vi "Sequencer Main - Copy.vi"() -> ()   [LabVIEW 2018]
uses:
  EDIT Sequencer V1/Ctl/MultiColumn Sequencer Table.ctl
  Examples - 32bit/SEQUENCER/SEQUENSER v10/Sequencer v10/Ctl/Devices INI Status.ctl
  PROJEKT/NIKO/Labview/Niko V4/FTDI SPI/Ctl/Sub Addr.ctl
  <vilib>/Utility/miscctls.llb/LVRowAndColumnUnsignedTypeDef.ctl
  <vilib>/Utility/miscctls.llb/LVRowAndColumnTypeDef.ctl
  EDIT Sequencer V1/Ctl/Test Step.ctl
  EDIT Sequencer V1/Ctl/Test Result.ctl
  Ctl Main/Global Variable.vi
  EDIT Sequencer V1/Ctl/Sequencer Array.vi
  <userlib>/_OpenG.lib/file/file.llb/File Exists - Scalar__ogtk.vi
  <vilib>/Utility/config.llb/Read Key (String).vi
  <vilib>/Utility/config.llb/Read Key (U32).vi
  <vilib>/Utility/config.llb/Read Key (Double).vi
  <vilib>/Utility/config.llb/Read Key (Boolean).vi
  <vilib>/measure/madcrms.llb/Basic Averaged DC-RMS for 1 Chan.vi
  <vilib>/printing/OpenHTMLReport.llb/Open HTML Report in Browser (Refnum).vi
  <vilib>/Utility/config.llb/Write Key (I32).vi
  <vilib>/regexp/Match Regular Expression.xnode
  <vilib>/Utility/NIReport.llb/NI_report.lvclass
  <vilib>/Utility/config.llb/NI_LVConfig.lvlib
  <vilib>/Utility/NIReport.llb/NI_ReportGenerationCore.lvlib
  <vilib>/measure/NI_MAPro.lvlib
panel:
  out "Pico Scope Correction":i32
  out "Handler":u32
  out "LogMsg":string
  in  "Sequenser":u16(ring) caption="SEQUENCER" items=["", "ADB-LMS (Dowble)", "ADB-LMS (Single)", "", "", ""]
  out "System Status":T1(ring)
  in  "Operator":u16(ring) caption="OPERATOR" items=["---", "Luc Switten", "Marius Dwornic", "Ion Popesku", "Serghei Nauc", "Test SNA"]
  out "Config":string
  out "Customer":string
  out "Under Test BOARD":string caption="Test BOARD"
  out "Nom New":dbl
  out "Max New":dbl
  out "Min New":dbl
  out "Nom Old":dbl
  out "Max Old":dbl
  out "Min Old":dbl
  in  "Application Quit":bool
  in  "Tab Control Main":T2(tab)
  in  "Debug":bool
  out "File Exist?":bool
  out "Device INI Config File Path":path
  out "Dev INI OK?":bool
  in  "Dev INI":bool
  out "Box Devices":T3
  out "System INI Config File":path
  in  "Enter STEP":u32 max=1000 step=1
  in  "Barcode\nDefault":bool
  out "Cnt False All":i32
  out "Cnt Pass All":i32
  out "Cnt Total All":i32
  in  "Reset cnt":bool
  in  "Auto\nSTART":bool
  out "RETEST":bool
  out "Test Time":string
  in  "Delay 1S":bool
  in  "Tab Control Msg":T4(tab)=enum."Scope"
  in  "Msg Str":string
  out "Switch Relay Modules":T5
  out "PowSupply - GET":T6 caption="GET" {"LowerLimit" format="%#.3g"; "Upper Limit" format="%#.3g"; "Power (W)" format="%#.3g"; "Current (mA)" format="%#.3g"; "Volt (V)" format="%#.3g"}
  out "PowSupply - SET":T7 caption="SET" {"Current Limit (A)" format="%#.3g"; "Volt (V)" format="%#.3g"}
  out "Max":dbl format="%#.3g"
  out "Nominal":dbl format="%#.3g"
  out "Min":dbl format="%#.3g"
  in  "DMM Measure Monitor":T8={"Mode"=enum."*****", "Measure"="23,45V"}
  out "Limits":cluster{dbl, dbl, dbl}(slide)={1.0972762645914398, 1.2996108949416343, 0.0} caption="Limits ***" scale=0.0..200.0 scale format="%^#_4g"
  in  "Serial CMD Mon":string
  in  "Correction":i32=-8 min=-200 max=200 step=1
  in  "F-Value":dbl=0.6499999999999999 min=-1.0 max=1.0 step=0.05
  out "Measure Ch-B":T9 {"MIN Vpp" format="%#.2f"; "MAX Vpp" format="%#_2f"; "PickToPick / 2" format="%#.2f"}
  out "Measure Ch-A":T10 {"MIN Vpp" format="%#.2f"; "MAX Vpp" format="%#.2f"; "PickToPoick / 2" format="%#.2f"}
  out "Channel A":cluster{i32, dbl, dbl[]}(graph)={0, 1.9999999949504854e-06, [0.0, 0.0, 0.0, 0.0, 0.0, 0.0, 0.0, 0.0, 0.0, 0.0, 0.0, 0.0, 0.0, 0.0, 0.0, 0.0, 0.0, 0.0, 0.0, 0.0, 0.0, 0.0, 0.0, 0.0, 0.0, 0.0, 0.0, 0.0, 0.0, 0.0, 0.0, 0.0, 0.0, 0.0, 0.0, 0.0, 0.0, 0.0, 0.0, 0.0, 0.0, 0.0, 0.0, 0.0, 0.0, 0.0, 0.0, 0.0, 0.0, 0.0, 0.0, 0.0, 0.0, 0.0, 0.0, 0.0, 0.0, 0.0, 0.0, 0.0, 0.0, 0.0, 0.0, 0.0, 0.0, 0.0, 0.0, 0.0, 0.0, 0.0, 0.0, 0.0, 0.0, 0.0, 0.0, 0.0, 0.0, 0.0, 0.0, 0.0, 0.0, 0.0, 0.0, 0.0, 0.0, 0.0, 0.0, 0.0, 0.0, 0.0, 0.0, 0.0, 0.0, 0.0, 0.0, 0.0, 0.0, 0.0, 0.0, 0.0, 0.0, 0.0, 0.0, 0.0, 0.0, 0.0, 0.0, 0.0, 0.0, 0.0, 0.0, 0.0, 0.0, 0.0, 0.0, 0.0, 0.0, 0.0, 0.0, 0.0, 0.0, 0.0, 0.0, 0.0, 0.0, 0.0, 0.0, 0.0, 0.0, 0.0, 0.0, 0.0, 0.0, 0.0, 0.0, 0.0, 0.0, 0.0, 0.0, 0.0, 0.0, 0.0, 0.0, 0.0, 0.0, 0.0, 0.0, 0.0, 0.0, 0.0, 0.0, 0.0, 0.0, 0.0, 0.0, 0.0, 0.0, 0.0, 0.0, 0.0, 0.0, 0.0, 0.0, 0.0, 0.0, 0.0, 0.0, 0.0, 0.0, 0.0, 0.0, 0.0, 0.0, 0.0, 0.0, 0.0, 0.0, 0.0, 0.0, 0.0, 0.0, 0.0, 0.0, 0.0, 0.0, 0.0, 0.0, 0.0, 0.0, 0.0, 0.0, 0.0, 0.0, 0.0, 0.0, 0.0, 0.0, 0.0, 0.0, 0.0, 0.0, 0.0, 0.0, 0.0, 0.0, 0.0, 0.0, 0.0, 0.0, 0.0, 0.0, 0.0, 0.0, 0.0, 0.0, 0.0, 0.0, 0.0, 0.0, 0.0, 0.0, 0.0, 0.0, 0.0, 0.0, 0.0, 0.0, 0.0, 0.0, 0.0, 0.0, 0.0, 0.0, 0.0, 0.0, 0.0, 0.0, 0.0, 0.0, 0.0, 0.0, 0.0, 0.0, 0.0, 0.0, 0.0, 0.0, 0.0, 0.0, 0.0, 0.0, 0.0, 0.0, 0.0, 0.0, 0.0, 0.0, 0.0, 0.0, 0.0, 0.0, 0.0, 0.0, 0.0, 0.0, 0.0, 0.0, 0.0, 0.0, 0.0, 0.0, 0.0, 0.0, 0.0, 0.0, 0.0, 0.0, 0.0, 0.0, 0.0, 0.0, 0.0, 0.0, 0.0, 0.0, 0.0, 0.0, 0.0, 0.0, 0.0, 0.0, 0.0, 0.0, 0.0, 0.0, 0.0, 0.0, 0.0, 0.0, 0.0, 0.0, 0.0, 0.0, 0.0, 0.0, 0.0, 0.0, 0.0, 0.0, 0.0, 0.0, 0.0, 0.0, 0.0, 0.0, 0.0, 0.0, 0.0, 0.0, 0.0, 0.0, 0.0, 0.0, 0.0, 0.0, 0.0, 0.0, 0.0, 0.0, 0.0, 0.0, 0.0, 0.0, 0.0, 0.0, 0.0, 0.0, 0.0, 0.0, 0.0, 0.0, 0.0, 0.0, 0.0, 0.0, 0.0, 0.0, 0.0, 0.0, 0.0, 0.0, 0.0, 0.0, 0.0, 0.0, 0.0, 0.0, 0.0, 0.0, 0.0, 0.0, 0.0, 0.0, 0.0, 0.0, 0.0, 0.0, 0.0, 0.0, 0.0, 0.0, 0.0, 0.0, 0.0, 0.0, 0.0, 0.0, 0.0, 0.0, 0.0, 0.0, 0.0, 0.0, 0.0, 0.0, 0.0, 0.0, 0.0, 0.0, 0.0, 0.0, 0.0, 0.0, 0.0, 0.0, 0.0, 0.0, 0.0, 0.0, 0.0, 0.0, 0.0, 0.0, 0.0, 0.0, 0.0, 0.0, 0.0, 0.0, 0.0, 0.0, 0.0, 0.0, 0.0, 0.0, 0.0, 0.0, 0.0, 0.0, 0.0, 0.0, 0.0, 0.0, 0.0, 0.0, 0.0, 0.0, 0.0, 0.0, 0.0, 0.0, 0.0, 0.0, 0.0, 0.0, 0.0, 0.0, 0.0, 0.0, 0.0, 0.0, 0.0, 0.0, 0.0, 0.0, 0.0, 0.0, 0.0, 0.0, 0.0, 0.0, 0.0, 0.0, 0.0, 0.0, 0.0, 0.0, 0.0, 0.0, 0.0, 0.0, 0.0, 0.0, 0.0, 0.0, 0.0, 0.0, 0.0, 0.0, 0.0, 0.0, 0.0, 0.0, 0.0, 0.0, 0.0, 0.0, 0.0, 0.0, 0.0, 0.0, 0.0, 0.0, 0.0, 0.0, 0.0, 0.0, 0.0, 0.0, 0.0, 0.0, 0.0, 0.0, 0.0, 0.0, 0.0, 0.0, 0.0, 0.0, 0.0, 0.0, 0.0, 0.0, 0.0, 0.0, 0.0, 0.0, 0.0, 0.0, 0.0, 0.0, 0.0, 0.0, 0.0, 0.0, 0.0, 0.0, 0.0, 0.0, 0.0, 0.0, 0.0, 0.0, 0.0, 0.0, 0.0, 0.0, 0.0, 0.0, 0.0, 0.0, 0.0, 0.0, 0.0, 0.0, 0.0, 0.0, 0.0, 0.0, 0.0, 0.0, 0.0, 0.0, 0.0, 0.0, 0.0, 0.0, 0.0, 0.0, 0.0, 0.0, 0.0, 0.0, 0.0, 0.0, 0.0, 0.0, 0.0, 0.0, 0.0, 0.0, 0.0, 0.0, 0.0, 0.0, 0.0, 0.0, 0.0, 0.0, 0.0, 0.0, 0.0, 0.0, 0.0, 0.0, 0.0, 0.0, 0.0, 0.0, 0.0, 0.0, 0.0, 0.0, 0.0, 0.0, 0.0, 0.0, 0.0, 0.0, 0.0, 0.0, 0.0, 0.0, 0.0, 0.0, 0.0, 0.0, 0.0, 0.0, 0.0, 0.0, 0.0, 0.0, 0.0, 0.0, 0.0, 0.0, 0.0, 0.0, 0.0, 0.0, 0.0, 0.0, 0.0, 0.0, 0.0, 0.0, 0.0, 0.0, 0.0, 0.0, 0.0, 0.0, 0.0, 0.0, 0.0, 0.0, 0.0, 0.0, 0.0, 0.0, 0.0, 0.0, 0.0, 0.0, 0.0, 0.0, 0.0, 0.0, 0.0, 0.0, 0.0, 0.0, 0.0, 0.0, 0.0, 0.0, 0.0, 0.0, 0.0, 0.0, 0.0, 0.0, 0.0, 0.0, 0.0, 0.0, 0.0, 0.0, 0.0, 0.0, 0.0, 0.0, 0.0, 0.0, 0.0, 0.0, 0.0, 0.0, 0.0, 0.0, 0.0, 0.0, 0.0, 0.0, 0.0, 0.0, 0.0, 0.0, 0.0, 0.0, 0.0, 0.0, 0.0, 0.0, 0.0, 0.0, 0.0, 0.0, 0.0, 0.0, 0.0, 0.0, 0.0, 0.0, 0.0, 0.0, 0.0, 0.0, 0.0, 0.0, 0.0, 0.0, 0.0, 0.0, 0.0, 0.0, 0.0, 0.0, 0.0, 0.0, 0.0, 0.0, 0.0, 0.0, 0.0, 0.0, 0.0, 0.0, 0.0, 0.0, 0.0, 0.0, 0.0, 0.0, 0.0, 0.0, 0.0, 0.0, 0.0, 0.0, 0.0, 0.0, 0.0, 0.0, 0.0, 0.0, 0.0, 0.0, 0.0, 0.0, 0.0, 0.0, 0.0, 0.0, 0.0, 0.0, 0.0, 0.0, 0.0, 0.0, 0.0, 0.0, 0.0, 0.0, 0.0, 0.0, 0.0, 0.0, 0.0, 0.0, 0.0, 0.0, 0.0, 0.0, 0.0, 0.0, 0.0, 0.0, 0.0, 0.0, 0.0, 0.0, 0.0, 0.0, 0.0, 0.0, 0.0, 0.0, 0.0, 0.0, 0.0, 0.0, 0.0, 0.0, 0.0, 0.0, 0.0, 0.0, 0.0, 0.0, 0.0, 0.0, 0.0, 0.0, 0.0, 0.0, 0.0, 0.0, 0.0, 0.0, 0.0, 0.0, 0.0, 0.0, 0.0, 0.0, 0.0, 0.0, 0.0, 0.0, 0.0, 0.0, 0.0, 0.0, 0.0, 0.0, 0.0, 0.0, 0.0, 0.0, 0.0, 0.0, 0.0, 0.0, 0.0, 0.0, 0.0, 0.0, 0.0, 0.0, 0.0, 0.0, 0.0, 0.0, 0.0, 0.0, 0.0, 0.0, 0.0, 0.0, 0.0, 0.0, 0.0, 0.0, 0.0, 0.0, 0.0, 0.0, 0.0, 0.0, 0.0, 0.0, 0.0, 0.0, 0.0, 0.0, 0.0, 0.0, 0.0, 0.0, 0.0, 0.0, 0.0, 0.0, 0.0, 0.0, 0.0, 0.0, 0.0, 0.0, 0.0, 0.0, 0.0, 0.0, 0.0, 0.0, 0.0, 0.0, 0.0, 0.0, 0.0, 0.0, 0.0, 0.0, 0.0, 0.0, 0.0, 0.0, 0.0, 0.0, 0.0, 0.0, 0.0, 0.0, 0.0, 0.0, 0.0, 0.0, 0.0, 0.0, 0.0, 0.0, 0.0, 0.0, 0.0, 0.0, 0.0, 0.0, 0.0, 0.0, 0.0, 0.0, 0.0, 0.0, 0.0, 0.0, 0.0, 0.0, 0.0, 0.0, 0.0, 0.0, 0.0, 0.0, 0.0, 0.0, 0.0, 0.0, 0.0, 0.0, 0.0, 0.0, 0.0, 0.0, 0.0, 0.0, 0.0, 0.0, 0.0, 0.0, 0.0, 0.0, 0.0, 0.0, 0.0, 0.0, 0.0, 0.0, 0.0, 0.0, 0.0, 0.0, 0.0, 0.0, 0.0, 0.0, 0.0, 0.0, 0.0, 0.0, 0.0, 0.0, 0.0, 0.0, 0.0, 0.0, 0.0, 0.0, 0.0, 0.0, 0.0, 0.0, 0.0, 0.0, 0.0, 0.0, 0.0, 0.0, 0.0, 0.0, 0.0, 0.0, 0.0, 0.0, 0.0, 0.0, 0.0, 0.0, 0.0, 0.0, 0.0, 0.0, 0.0, 0.0, 0.0, 0.0, 0.0, 0.0, 0.0]}
  out "Channel B":cluster{i32, dbl, dbl[]}(graph)={0, 1.9999999949504854e-06, [0.0, 0.03891109958189642, 0.03891109958189642, 0.0, 0.03891109958189642, 0.03891109958189642, 0.03891109958189642, 0.0, 0.0, 0.03891109958189642, 0.03891109958189642, 0.03891109958189642, 0.03891109958189642, -0.03891109958189642, 0.0, 0.0, 0.0, 0.03891109958189642, 0.0, 0.0, 0.03891109958189642, 0.0, 0.03891109958189642, 0.0, 0.0, 0.0, 0.0, 0.03891109958189642, 0.03891109958189642, 0.0, -0.03891109958189642, 0.03891109958189642, 0.0, 0.03891109958189642, 0.03891109958189642, 0.03891109958189642, 0.0, 0.0, 0.03891109958189642, 0.0, 0.0, 0.03891109958189642, 0.03891109958189642, 0.0, 0.0, 0.03891109958189642, 0.0, 0.03891109958189642, 0.0, 0.0, 0.0, 0.03891109958189642, 0.03891109958189642, 0.0, 0.0, 0.0, 0.03891109958189642, 0.03891109958189642, 0.0, 0.0, 0.03891109958189642, 0.0, 0.0, -0.03891109958189642, 0.03891109958189642, 0.0, 0.0, 0.0, 0.0, 0.03891109958189642, 0.0, 0.0, 0.03891109958189642, 0.0, 0.03891109958189642, -0.03891109958189642, 0.0, 0.0, 0.03891109958189642, 0.0, 0.03891109958189642, 0.03891109958189642, 0.0, 0.0, 0.03891109958189642, 0.0, 0.03891109958189642, 0.0, 0.0, 0.0, 0.0, 0.03891109958189642, 0.0, 0.0, 0.03891109958189642, 0.03891109958189642, 0.0, 0.0, 0.0, 0.03891109958189642, 0.0, 0.0, 0.0, 0.0, 0.0, 0.0, 0.0, 0.0, 0.0, 0.0, 0.0, 0.03891109958189642, 0.0, 0.03891109958189642, 0.03891109958189642, 0.0, 0.03891109958189642, 0.03891109958189642, 0.0, 0.03891109958189642, 0.0, 0.0, 0.0, 0.03891109958189642, 0.03891109958189642, 0.0, 0.0, 0.0, 0.0, 0.0, 0.03891109958189642, 0.0, 0.03891109958189642, 0.0, 0.0, 0.03891109958189642, 0.03891109958189642, 0.0, 0.0, 0.0, 0.03891109958189642, 0.03891109958189642, 0.0, 0.0, 0.03891109958189642, 0.0, 0.0, 0.03891109958189642, 0.0, 0.0, 0.0, 0.03891109958189642, 0.0, 0.03891109958189642, 0.03891109958189642, 0.03891109958189642, 0.03891109958189642, 0.03891109958189642, 0.0, 0.0, 0.0, 0.03891109958189642, 0.03891109958189642, 0.03891109958189642, 0.03891109958189642, 0.03891109958189642, 0.0, 0.03891109958189642, 0.0, 0.0, 0.0, 0.03891109958189642, 0.0, 0.03891109958189642, 0.0, 0.0, 0.0, 0.0, 0.03891109958189642, 0.0, 0.0, 0.03891109958189642, 0.0, 0.03891109958189642, 0.03891109958189642, 0.0, 0.03891109958189642, 0.0, 0.03891109958189642, 0.03891109958189642, 0.03891109958189642, 0.03891109958189642, 0.0, 0.03891109958189642, 0.03891109958189642, 0.0, 0.0, 0.03891109958189642, 0.03891109958189642, 0.03891109958189642, 0.03891109958189642, 0.0, 0.0, 0.0, 0.0, 0.03891109958189642, 0.0, 0.03891109958189642, 0.0, 0.03891109958189642, 0.0, 0.0, 0.0, 0.03891109958189642, 0.03891109958189642, 0.0, 0.0, 0.0, 0.0, 0.03891109958189642, 0.0, 0.0, 0.0, 0.0, 0.03891109958189642, 0.03891109958189642, 0.03891109958189642, 0.0, 0.03891109958189642, 0.0, 0.0, 0.0, 0.03891109958189642, 0.03891109958189642, 0.03891109958189642, 0.03891109958189642, 0.0, 0.0, 0.0, 0.0, 0.03891109958189642, 0.03891109958189642, 0.03891109958189642, 0.03891109958189642, 0.0, 0.0, 0.0, 0.0, 0.0, 0.0, 0.03891109958189642, 0.0, 0.0, 0.0, -0.03891109958189642, 0.0, 0.0, 0.03891109958189642, 0.03891109958189642, 0.0, 0.0, 0.03891109958189642, 0.03891109958189642, 0.0, 0.0, 0.03891109958189642, -0.03891109958189642, 0.03891109958189642, 0.03891109958189642, 0.0, 0.0, 0.0, 0.0, 0.03891109958189642, 0.03891109958189642, 0.0, 0.03891109958189642, 0.0, 0.0, 0.0, 0.0, 0.0, 0.0, 0.0, 0.03891109958189642, 0.03891109958189642, 0.0, 0.03891109958189642, 0.03891109958189642, 0.0, 0.0, 0.0, 0.03891109958189642, 0.0, 0.0, 0.0, 0.0, 0.0, 0.0, 0.0, 0.0, 0.0, 0.0, 0.03891109958189642, 0.0, 0.0, 0.0, 0.0, 0.0, 0.0, 0.0, 0.03891109958189642, 0.0, 0.0, 0.0, 0.0, 0.0, 0.0, 0.0, 0.0, 0.0, 0.03891109958189642, 0.0, 0.0, 0.0, 0.03891109958189642, 0.0, 0.03891109958189642, 0.0, 0.03891109958189642, 0.03891109958189642, 0.0, 0.03891109958189642, 0.0, 0.03891109958189642, 0.0, 0.03891109958189642, 0.0, 0.03891109958189642, 0.0, -0.03891109958189642, 0.0, 0.0, 0.0, 0.0, 0.0, 0.03891109958189642, 0.0, 0.03891109958189642, 0.0, 0.03891109958189642, 0.03891109958189642, 0.0, 0.0, 0.0, 0.03891109958189642, 0.0, 0.03891109958189642, 0.03891109958189642, 0.0, 0.0, 0.0, 0.0, 0.0, 0.0, 0.03891109958189642, 0.03891109958189642, 0.0, 0.0, 0.0, 0.0, 0.0, 0.0, 0.0, -0.03891109958189642, 0.03891109958189642, 0.0, 0.03891109958189642, 0.03891109958189642, 0.0, 0.0, 0.03891109958189642, 0.0, 0.03891109958189642, 0.0, 0.0, 0.03891109958189642, 0.03891109958189642, 0.03891109958189642, 0.0, 0.0, 0.03891109958189642, 0.03891109958189642, 0.03891109958189642, 0.0, 0.0, 0.0, 0.0, 0.0, 0.0, 0.0, 0.0, 0.03891109958189642, 0.0, 0.03891109958189642, 0.0, 0.0, 0.03891109958189642, 0.03891109958189642, 0.03891109958189642, 0.0, 0.0, 0.0, 0.0, 0.03891109958189642, -0.03891109958189642, 0.03891109958189642, 0.0, 0.03891109958189642, 0.03891109958189642, 0.0, 0.0, 0.03891109958189642, 0.0, 0.0, 0.03891109958189642, 0.0, 0.0, 0.0, -0.03891109958189642, 0.03891109958189642, 0.03891109958189642, 0.03891109958189642, 0.03891109958189642, 0.03891109958189642, 0.03891109958189642, 0.03891109958189642, 0.0, 0.0, 0.0, 0.0, 0.0, 0.0, 0.0, 0.0, 0.03891109958189642, 0.03891109958189642, 0.0, 0.0, 0.0, 0.03891109958189642, 0.03891109958189642, 0.0, 0.0, 0.0, 0.03891109958189642, 0.0, 0.0, 0.0, 0.0, 0.0, 0.03891109958189642, 0.03891109958189642, 0.03891109958189642, 0.0, 0.0, 0.0, 0.03891109958189642, 0.0, 0.03891109958189642, 0.03891109958189642, 0.03891109958189642, 0.03891109958189642, 0.0, 0.03891109958189642, 0.0, 0.0, 0.0, 0.03891109958189642, 0.0, 0.0, 0.0, 0.0, 0.0, 0.03891109958189642, 0.03891109958189642, 0.03891109958189642, 0.0, 0.0, 0.03891109958189642, 0.03891109958189642, -0.03891109958189642, 0.0, 0.03891109958189642, 0.0, 0.0, 0.0, 0.03891109958189642, 0.03891109958189642, 0.0, 0.0, 0.0, 0.0, 0.0, 0.0, 0.0, 0.0, 0.03891109958189642, 0.03891109958189642, 0.03891109958189642, 0.0, 0.03891109958189642, 0.03891109958189642, 0.03891109958189642, 0.0, 0.03891109958189642, 0.0, 0.0, 0.03891109958189642, 0.0, 0.03891109958189642, 0.0, 0.0, 0.0, 0.0, 0.0, 0.0, 0.0, 0.0, 0.03891109958189642, 0.0, 0.03891109958189642, 0.03891109958189642, 0.03891109958189642, 0.03891109958189642, 0.0, 0.03891109958189642, 0.03891109958189642, 0.0, 0.0, 0.0, 0.03891109958189642, 0.0, 0.03891109958189642, 0.03891109958189642, 0.0, 0.0, 0.0, 0.0, 0.0, 0.0, 0.03891109958189642, 0.0, 0.0, 0.03891109958189642, 0.03891109958189642, 0.0, 0.0, 0.0, 0.0, 0.03891109958189642, 0.03891109958189642, 0.0, 0.0, 0.0, 0.03891109958189642, 0.0, 0.0, 0.0, 0.0, 0.03891109958189642, 0.0, 0.0, 0.0, 0.0, 0.03891109958189642, 0.03891109958189642, 0.03891109958189642, 0.0, 0.0, 0.0, 0.03891109958189642, 0.03891109958189642, 0.03891109958189642, 0.0, 0.03891109958189642, 0.0, 0.0, 0.0, 0.0, 0.03891109958189642, 0.0, 0.03891109958189642, 0.0, 0.0, 0.03891109958189642, 0.03891109958189642, 0.03891109958189642, 0.0, 0.0, 0.03891109958189642, 0.0, 0.0, 0.03891109958189642, 0.0, 0.0, 0.03891109958189642, 0.03891109958189642, 0.0, 0.03891109958189642, 0.0, 0.0, 0.0, 0.0, 0.0, 0.0, 0.0, 0.03891109958189642, 0.03891109958189642, 0.0, 0.03891109958189642, 0.0, 0.03891109958189642, 0.0, 0.0, 0.03891109958189642, 0.03891109958189642, 0.0, 0.03891109958189642, 0.03891109958189642, -0.03891109958189642, 0.03891109958189642, 0.0, 0.03891109958189642, 0.0, -0.03891109958189642, 0.0, 0.03891109958189642, 0.03891109958189642, 0.03891109958189642, 0.0, 0.0, 0.0, 0.0, 0.0, 0.03891109958189642, 0.0, 0.03891109958189642, 0.0, 0.0, 0.0, 0.0, 0.03891109958189642, 0.0, 0.03891109958189642, 0.0, 0.03891109958189642, 0.0, 0.03891109958189642, 0.0, 0.03891109958189642, 0.0, 0.03891109958189642, 0.0, 0.03891109958189642, 0.0, 0.03891109958189642, 0.0, 0.0, 0.03891109958189642, 0.0, 0.03891109958189642, 0.0, 0.0, 0.0, 0.0, 0.0, 0.0, 0.03891109958189642, 0.0, 0.0, 0.03891109958189642, 0.0, 0.03891109958189642, 0.0, 0.0, 0.0, 0.0, 0.0, 0.03891109958189642, 0.03891109958189642, 0.0, -0.03891109958189642, 0.0, 0.03891109958189642, 0.0, 0.0, 0.03891109958189642, 0.03891109958189642, 0.0, 0.03891109958189642, 0.03891109958189642, 0.03891109958189642, 0.0, 0.03891109958189642, 0.03891109958189642, 0.03891109958189642, 0.0, 0.0, 0.03891109958189642, 0.03891109958189642, 0.03891109958189642, 0.03891109958189642, 0.0, 0.03891109958189642, 0.0, 0.0, 0.0, 0.03891109958189642, 0.03891109958189642, 0.03891109958189642, 0.0, 0.0, 0.03891109958189642, 0.0, 0.0, 0.03891109958189642, 0.0, 0.03891109958189642, 0.0, 0.03891109958189642, 0.0, 0.03891109958189642, 0.0, 0.0, 0.0, 0.0, 0.0, 0.03891109958189642, 0.0, 0.0, 0.0, 0.0, 0.03891109958189642, 0.0, 0.0, 0.0, 0.0, 0.0, 0.0, 0.0, 0.0, 0.0, 0.0, 0.0, 0.0, 0.03891109958189642, -0.03891109958189642, 0.03891109958189642, 0.0, 0.07782219916379284, 0.03891109958189642, 0.0, 0.03891109958189642, 0.0, 0.03891109958189642, 0.0, 0.03891109958189642, 0.03891109958189642, 0.03891109958189642, 0.03891109958189642, 0.03891109958189642, 0.0, 0.0, 0.03891109958189642, 0.0, 0.03891109958189642, 0.0, 0.0, 0.0, 0.0, 0.0, 0.03891109958189642, 0.03891109958189642, 0.0, 0.0, 0.03891109958189642, 0.03891109958189642, 0.03891109958189642, 0.0, 0.03891109958189642, 0.0, 0.03891109958189642, 0.03891109958189642, 0.0, 0.03891109958189642, -0.03891109958189642, 0.0, 0.03891109958189642, 0.0, 0.03891109958189642, 0.03891109958189642, 0.0, 0.03891109958189642, 0.0, 0.0, 0.0, 0.0, 0.0, 0.03891109958189642, 0.0, 0.0, 0.0, 0.03891109958189642, 0.07782219916379284, 0.0, 0.03891109958189642, 0.0, 0.0, 0.03891109958189642, 0.0, 0.0, 0.03891109958189642, 0.0, 0.03891109958189642, 0.0, 0.03891109958189642, 0.0, 0.0, 0.03891109958189642, 0.0, 0.0, 0.03891109958189642, 0.0, 0.03891109958189642, 0.0, 0.0, 0.0, 0.03891109958189642, 0.03891109958189642, 0.03891109958189642, -0.03891109958189642, 0.03891109958189642, 0.03891109958189642, 0.03891109958189642, 0.03891109958189642, 0.0, 0.0, 0.0, 0.0, 0.0, 0.03891109958189642, 0.0, 0.0, 0.0, 0.0, 0.03891109958189642, 0.0, 0.0, 0.0, 0.03891109958189642, 0.03891109958189642, 0.0, 0.0, 0.03891109958189642, 0.0, 0.03891109958189642, 0.03891109958189642, 0.0, 0.0, 0.0, 0.03891109958189642, 0.03891109958189642, 0.0, 0.03891109958189642, 0.0, 0.0, 0.0, 0.03891109958189642, 0.03891109958189642, 0.0, 0.0, 0.03891109958189642, 0.03891109958189642, 0.03891109958189642, 0.03891109958189642, 0.03891109958189642, 0.03891109958189642, 0.03891109958189642, 0.03891109958189642, 0.0, 0.0, 0.03891109958189642, 0.03891109958189642, 0.0, 0.0, 0.03891109958189642, 0.03891109958189642, 0.0, 0.03891109958189642, 0.0, 0.03891109958189642, 0.03891109958189642, 0.0, 0.03891109958189642, 0.0, 0.0, 0.0, 0.0, 0.03891109958189642, 0.0, 0.0, 0.03891109958189642, 0.03891109958189642, 0.0, 0.07782219916379284, 0.0, 0.0, 0.03891109958189642, 0.0, 0.03891109958189642, 0.0, 0.03891109958189642, 0.03891109958189642, 0.0, 0.0, 0.0, 0.0, 0.0, 0.03891109958189642, 0.03891109958189642, 0.03891109958189642, 0.03891109958189642, 0.0, 0.0, 0.03891109958189642, 0.0, 0.0, 0.03891109958189642, 0.0, 0.0, 0.03891109958189642, 0.03891109958189642, 0.03891109958189642, 0.0, 0.03891109958189642, 0.0, 0.0, 0.0, 0.03891109958189642, 0.03891109958189642, 0.03891109958189642, 0.03891109958189642, 0.03891109958189642, 0.0, 0.0, 0.0, 0.0, 0.0, 0.0, 0.03891109958189642, 0.03891109958189642, 0.0, 0.03891109958189642, 0.03891109958189642, 0.0, 0.03891109958189642, -0.03891109958189642, 0.03891109958189642, 0.0, 0.03891109958189642, 0.0, -0.03891109958189642, 0.0, 0.03891109958189642, 0.0, 0.0, 0.03891109958189642, 0.03891109958189642, 0.03891109958189642, 0.03891109958189642, 0.03891109958189642, 0.07782219916379284, 0.03891109958189642, 0.0, 0.03891109958189642, 0.0, 0.03891109958189642, 0.0, 0.03891109958189642, 0.03891109958189642, 0.03891109958189642, 0.03891109958189642, 0.0, 0.0, 0.0, 0.03891109958189642, 0.0, 0.03891109958189642, 0.03891109958189642]}
  in  "Delay":u16=2 max=10 step=1
  in  "Tab Edit/Run":enum32{"Edit", "Run"}(tab)
  in  "Test Squencer Edit":T11
  in  "Test Sequencer Run":T11
  in  "Dig-IN Claster":T12
  in  "Break Point Line":u32
  out "Sys Err":bool
  in  "Report Auto":bool=TRUE
  in  "Break On First Err":bool=TRUE caption="Break On\n3x First Err"
  in  "Button Create Report":bool
  in  "Abort Test":bool
  in  "Run Test":bool
  in  "Button Retest":bool
  in  "Button Next Step":bool caption="Next Step"
  in  "Debugging":bool
  in  "Edit Sequenser":bool
  out "Cnt False":i32
  out "Cnt Pass":i32
  out "Cnt Total":i32
  out "Gen Test Status":bool
  in  "Load Sequenser":bool
  in  "Message":string="..."
  in  "Barcode":string="ADB-12345"
  out "Date Time":string
  in  "Auto\nRestart":u16=1 min=1 max=99
  out "Restart Cnt":u16
  out "Auto\nReStart":bool
  in  "WebBrowser":refnum<k7>(container)
  in  "Open in Default IE":bool
  out "Help":string="GPIO-Out Set RELAY Modules: \n(Step-Id = 10)                        std_logic_vector(9 downto 0) use (9 downto 0)\n      0>1>d:1                          --set single decimal channel ;\n      0>1>b:0000110001       -- set binary multiple channels ;\n      0>1>s:0000000011        -- Set  binary (only 1 channels) ;\n      0>1>r:0000000011        -- Reset  binary (only 1 channels) ;\n      --option 'Togle Channel' not in use\n\nGPIO-Out Set SYSTEM: \n(Step-Id = 11)                           std_logic_vector(9 downto 0) use (3 downto 0)\n      0>1>b:0000110001        -- set binary multiple channels ;\n\nRESET Modules ( (GPIO->ON) >> (GPIO->OFF) )\n(Step-Id = 12)\n    0>1>rst:0000000011>250>1000        -- reset 0>1>channel:xx>Delay(Active)>Delay(Passive)\n\nDELAY (mS)\n(Step-Id = 13)\n    750                                     --Delay (750mS)\n\nPOWER SUPPLY (BK9201) \n   1- Set (Step-Id = 15)\n        57,0>0,2>ON           --set Volt>Current>ON/OFF\n\n   2- Get (Step-Id = 16)\n       Volt?\n       Current?\n       Power?\n\nDMM bk5492C\n(Step-Id = 20)                   <measure DMM-DC Volt>\n       V-DC>0                   --Auto Range\n       V-DC>0,1                --Manual Range (0,1 1 10 100 1000)V\n       -----------------------------------------------------------------------------------------------\n                                          <measure DMM-AC Volt>\n       V-AC>0                   --Auto Range\n       V-AC>0,1                --Manual Range (0,1 1 10 100 750)V\n       -----------------------------------------------------------------------------------------------\n                                                               <measure DMM-Resistors 2x Wires>\n       R-2W>0                 --Auto Range\n           R-2W>1M              --Manual Range (10, 100, 1K, 10K, 100K, 1M, 10M, 100M)\n       ----------------------------------------------------------------------------------------------- \n                                                               <measure DMM-Resistors 4x Wires>\n       R-4W>0                 --Auto Range\n           R-4W>10K             --Manual Range (10, 100, 1K, 10K, 100K, 1M, 10M, 100M)  \n       -----------------------------------------------------------------------------------------------\n\n      >false:100:2       --in case of a FALSE, repeat test 2x times, gump to step100\n\nFLASH ADB\n(Step-Id = 70)\n       adb_flash.bat      --xxxx.bat -name of bat file, location at ..\\FLASH\n\nSERIAL CMD (RS232)\n(Step-Id = 60) \n       >>open;<firmware version>      --Open Serial COM and check firmware version\n\n      >false:100:2       --in case of a FALSE, repeat test 2x times, gump to step100\n\n\nBLUETOOTH (u-blox)\n(Step-Id = 40)                   <Connect To ADB Bloetooth Interfice>\n\nRFID (Arduino & Sparkfun uno)\n(Step-Id = 45)                   <Connect To ADB RFID Interfice>\n      >false:100:2       --in case of a FALSE, repeat test 2x times, gump to step100\n\nRFID (Arduino & Sparkfun uno)\n(Step-Id = 46)                   <Connect To ADB RFID Interfice>\n      >false:100:2       --in case of a FALSE, repeat test 2x times, gump to step100\n\nPicoScope (SET)\n(Step-Id = 51)             --Set PicoScope (Time Aut = 2000mS)\n      A>8000>1000           Channel <A, B> ; Sampels ;TimeBase\n\nPicoScope (GET)\n(Step-Id = 51)             --Read PicoScope DATA\n      A>>false:100:2            Channel <A, B> ; Sampels ;TimeBase\n                                          --if FALSE, repeat test 2x times, gump to step100\n\n(Step-Id = 52)             --Read PicoScope (Time Aut = 2000mS)\n      B>false:46:3               Channel <A, B> if FALSE, goto step <46>, retry <3> times \n\n(Step-Id = 53)                     --Read PicoScope \"Positive / Negative Measurement\" (Time Aut = 2000mS)\n      B>Positive>false:46:3               Channel <A, B> if FALSE, goto step <46>, retry <3> times \n      B>Negative\n\n\n\n\n\n\n\n   "
  # "ELETEST-Ro Test SEQUENCER"
  # "Elemaster Romania"
  # "ver 3,0"
  # "TEST Report STATUS"
  # "Dig Sys Input"
  # "Fixture Closed"
  # "Barcode"
  # "Stop"
  # "Run"
  # "TOTAL:"
  # "Sequencer / Debugging"
  # "PASS:"
  # "FALSE:"
  # "1"
  # "2"
  # "3"
  # "4"
  # "5"
  # "6"
  # "7"
  # "8"
  # "9"
  # "10"
  # "Ch-A"
  # "Ch-B"
  # "DMM Measure Mode"
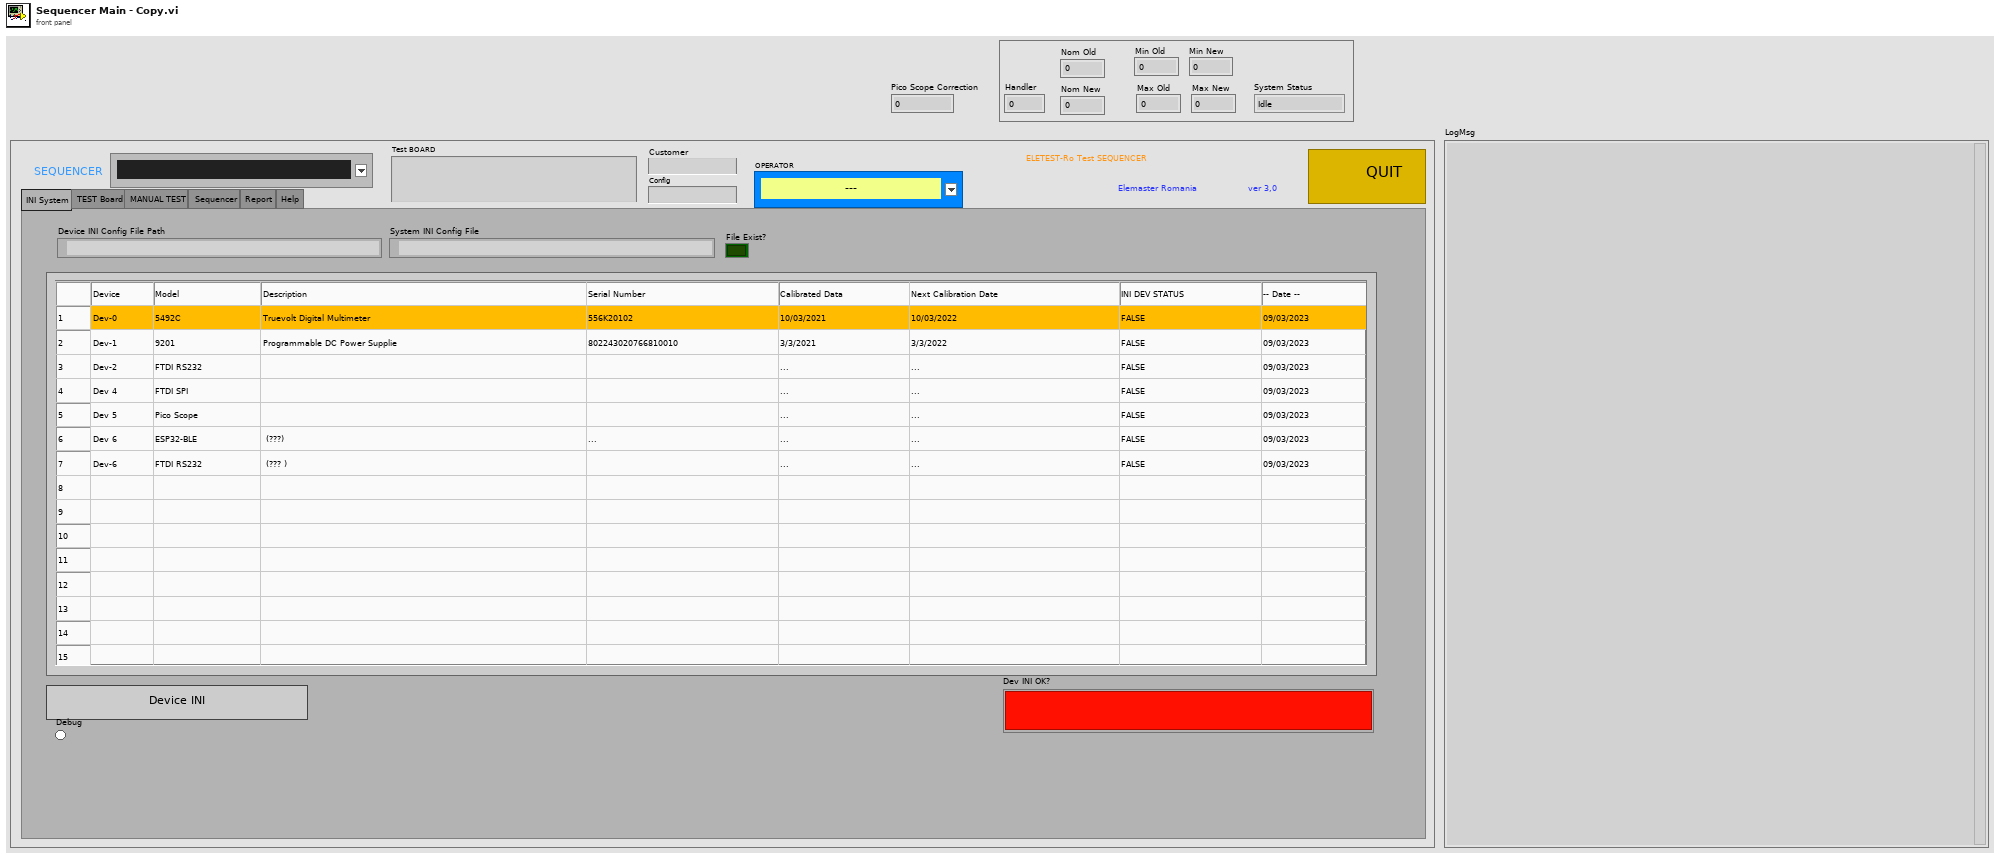
[diagram p1: front panel]
types:
  T1 = enum16{"Idle", "INI System", "INI Devices", "START Sequencer", "INI Secuencer", "Run Sequencer", "STOP Sequencer", "Report Generation", "Test Load Monitor", "QUIT"}
  T2 = enum32{"INI System", "TEST Board", "MANUAL TEST", "Sequencer ", "Report", "Help"}
  T3 = typedef "Devices INI Status.ctl" = i32
  T4 = enum32{"Msg", "Settings", "PowSupply", "DMM", "Serial", "Scope", "Bluetooth"}
  T5 = cluster{"SW 0":bool[], "SW 1":bool[], "SW 2":bool[], "SW 3":bool[], "SW 4":bool[], "SW 5":bool[], "SW 6":bool[], "SW 7":bool[], "Main Power Supplay ON/OFF":bool, "BASE":bool[][]}
  T6 = cluster{"Volt (V)":dbl, "Current (mA)":dbl, "Power (W)":dbl, "Upper Limit":dbl, "LowerLimit":dbl}
  T7 = cluster{"Volt (V)":dbl, "Current Limit (A)":dbl, "ON/OFF":bool}
  T8 = cluster{"Mode":enum16{"*****", "Voltage - DC", "Voltage - AC", "Current - DC", "Current - AC", "Diode", "Resistans 2-Wire", "Resistans 4-Wire", "Capasitor"}, "Measure":string}
  T9 = cluster{"PickToPick / 2":dbl, "MAX Vpp":dbl, "MIN Vpp":dbl}
  T10 = cluster{"PickToPoick / 2":dbl, "MAX Vpp":dbl, "MIN Vpp":dbl}
  T11 = typedef "MultiColumn Sequencer Table.ctl" = i32
  T12 = cluster{"Stop":bool, "Fixture Close":bool, "digIn 3":bool, "digIn 4":bool, "Run":bool}
  T13 = typedef "Semaphore RefNum" = refnum<k1>
  T14 = typedef "LVRowAndColumnUnsignedTypeDef.ctl" = cluster{"Row":u32, "Column":u32}
  T15 = typedef "LVRowAndColumnTypeDef.ctl" = cluster{"Row":i32, "Column":i32}
  T16 = typedef "Test Step.ctl" = cluster{"Step ID":u16, "Step Description":string, "Step Type":u16, "Test Values":cluster{"Numeric Value":dbl, "Str Value":string, "Boolean Value":bool, "Upper Limit":dbl, "Lower Limit":dbl}, "Parameters":string, "Run/Skip":bool, "Test Result":T17, "Report":bool, "Measure Units":string}
  T17 = typedef "Test Result.ctl" = enum16{"Idle", "PASS", "FALSE"}
  T18 = enum8{"Enabled", "Disabled", "Disabled and Grayed Out"}
  T19 = typedef "NI_LVConfig.lvlib/Config Data RefNum.ctl" = refnum<k1>
  T20 = typedef "Sub Addr.ctl" = u16
  T21 = enum32{"Msg", "Settings", "PowSupply", "DMM", "Serial", "Scope"}
  T22 = cluster{"ClockRate":u32, "LatencyTimer":u8, "configOptions 24-31":i8, "configOptions 16-23":i8, "configOptions 8-15":i8, "configOptions 0-7":u32, "Pin":u32, "reserved":u16}
  T23 = enum16{"Set Decimal", "Set Binary", "Set Channels", "Reset Channels"}
  T24 = enum16{"Set Decimal", "Set Binary", "Set Channels", "Reset Channels", "Togle Channel"}
  T25 = enum16{"*****", "Voltage - DC", "Voltage - AC", "Current - DC", "Current - AC", "Diode", "Resistans 2-Wire", "Resistans 4-Wire", "Capasitor"}
  T26 = cluster{"Enabled":bool, "Coupling":i16, "Range":u16, "Analogue Offset":sgl}
  T27 = cluster{"preTriggerSamples":u32, "postTriggerSamples":u32, "timebase":u32, "Down-Sample Mode":i32, "Down Sample Ratio":u32, "Oversample":i16}
  T28 = cluster{"Trigger Enabled":bool, "Trigger Source":enum16{"Channel A", "Channel B", "Channel C", "Channel D", "Ext."}, "Trigger Threshold (Volts)":dbl, "Trigger Direction":u16, "Trigger Delay (samples)":u32, "Auto Trigger Time (ms)":i16}
  T29 = cluster{"Peak-to-Peak Voltage (microvolts)":u32, "Offset Voltage (microvolts)":i32, "Wave Type":i16, "Sweep Type":i32, "Shots":u32, "Sweeps":u32, "Trigger Type":i32, "Trigger Source":i32, "Ext. Threshold (ADC count)":i16, "White Noise":bool}
  T30 = cluster{"Start Frequency":dbl, "Stop Frequency":dbl, "Increment":dbl, "Dwell Time (seconds)":dbl}
  T31 = enum16{"Standard Report", "HTML", "Word", "Excel"}
  T32 = cluster{"top":dbl, "left":dbl, "right":dbl, "bottom":dbl}
  T33 = typedef "LVStringsAndValuesArrayTypeDef_U16.ctl" = cluster{"String":string, "Value":u16}[]
  T34 = typedef "Serial_VISA.ctl" = cluster{"VISA resource name":string, "Vendor":string, "SerialNumber":string, "CalibrationTime":string, "Dev Ok":bool, "Model":string, "Next CalibrationTime":string}
  T35 = cluster{"Driver Version":string, "USB Version":string, "Hardware":string, "Variant":string, "Batch and Serial":string, "Cal Date":string, "Kernel Version":string, "Digital HW Version":string, "Analogue HW Version":string, "Firmware 1":string, "Firmware 2":string, "MSO":bool, "Number of Channels":i16}
  T36 = cluster{"Lower Limit":dbl, "Upper Limit":dbl, "Numeric Value":dbl}
  T37 = cluster{"Lower Limit":dbl, "Upper Limit":dbl, "Result Value":dbl}
diagram:
  n1 = in-place {
    in-place-border: [w7] -> w1
    in-place-border: [w11] -> w3
    in-place-border: [w10] -> w2
    in-place-border: [w9] -> w5
    in-place-border: [w8] -> w4
    w7 = errorcluster {"status"=FALSE, "code"=0, "source"=""} ("error in (no error)")
    # "INI Section"
    n2 = Initialize Array(w7, 20 ("dimension size")) -> (w14:errorcluster[])
    n3 = global write "Global Variable.vi" "System Status"(T1."INI System" ("System Status")) -> ()
    n4 = global write "Global Variable.vi" "Array Errors"(w14) -> ()
    n5 = Obtain Queue(element data type=0, error in (no error)=w7) -> (queue out=w11:refnum<queue>, error out=w10:errorcluster)  [unwired: 3 in, 1 out]
    n6 = call <vilib>:"Obtain Semaphore Reference.vi"("error in (no error)"=w7) -> ("error out"=w9:errorcluster, "semaphore"=w8:T13)  [unwired: 4 in, 1 out]
  }
  n7 = in-place {
    in-place-border: w1 -> [w32]
    # "Read INI System File"
    # "Edit Sequencer Sub Pannel"
    n8 = vi-ref "Edit Saquencer Array.vi"() -> (w33:refnum<vi>)
    n9 = property class="VI"(reference=w33) -> ("Path"=w31:path)  [unwired: 1 in, 2 out]
    n10 = Open VI Reference(type specifier VI Refnum (for type only)=refnum<vi> refnum, vi path=w31, error in (no error)=w32) -> (vi reference=w20:refnum<vi>, error out=w22:errorcluster)  [unwired: 3 in]
    n11 = call <vilib>:"Application Directory.vi"() -> ("Application Directory"=w17:path)
    n12 = invoke on="Sub Panel Sequenser Edit" class="SubPnl" method="Insert VI"(error in=w22, "VI Ref"=w20) -> (error out=w21:errorcluster)  [unwired: 2 in, 3 out]
    n13 = Build Path(base path=w17, name or relative path="INI\\SysConfig.ini") -> (appended path=w15:path)
    n14 = call-by-ref "?"(reference=w20, error in=w21, "Sys Ini Path"=w15) -> (reference out=w18:refnum<vi>, error out=w19:errorcluster)  [unwired: 11 in]
    n15 = while {
      tunnel: [w35] -> w30
      tunnel: w18 -> [w35]
      stop <- FALSE stop-if-true
      n16 = Wait (ms)(milliseconds to wait=u32 250) -> ()  [unwired: 1 out]
    }
    n17 = invoke class="VI (strict)" method="FP.Close"(reference=w30, error in=w19) -> (reference out=w29:refnum<vi>, error out=w28:errorcluster)  [unwired: 1 in, 1 out]
    n18 = global read "Global Variable.vi" "Array Errors"() -> (w27:errorcluster[])
    n19 = Close Reference(reference=w29, error in (no error)=w28) -> (error out=w25:errorcluster)
    n20 = Replace Array Subset(array=w27, new element=w25, index=0) -> (w26:errorcluster[])
    n21 = global write "Global Variable.vi" "Array Errors"(w26) -> ()
  }
  n22 = in-place {
    in-place-border: w3 -> [w38]
    in-place-border: w2 -> [w37]
    n23 = while {
      tunnel: w38 -> [w40]
      tunnel: w37 -> [w39]
      stop <- FALSE stop-if-true
      # "DATA/TIME & Key Board (Events)"
      n24 = event shown="[3] \"Application Quit\": Value Change" {
        selector: _ -> [_ _ _ _ _ _ _ _ _ _ _ _ _ _ _]
        dyn-events: _ -> [_ _ _ _ _ _ _ _ _ _ _ _ _ _ _]
        timeout: 1000 -> [_ _ _ _ _ _ _ _ _ _ _ _ _ _ _]
        tunnel: w40 -> [_ _ _ w123 w152 _ _ _ _ w263 _ w338 w352 _ _]
        tunnel: w39 -> [_ _ _ w122 w151 _ _ _ _ w262 _ w337 w351 _ _]
        event Timeout {
          n25 = event-data() -> ()  [unwired: 1 in, 3 out]
          n26 = flat-sequence {
            tunnel: "Debugging" -> [w44]
            frame #0 {
              n27 = case shown="False" w44 {
                frame False {
                  w69 = T18."Disabled and Grayed Out" ("Disabled")
                  n28 = global read "Sequencer Array.vi" "SEQUENCER Array"() -> (w67:T16[])
                  n29 = property on="Break Point Line" class="DigNum (strict)"("Value"=u32 0 ("Break Point Cnt")) -> ()  [unwired: 2 in, 2 out]
                  n30 = local read "Break Point Line"() -> (w64:u32)
                  n31 = Array Size(array=w67) -> (size(s)=w66:i32)
                  n32 = Initialize Array(0, w66) -> (w61:i32[])
                  n33 = Replace Array Subset(array=w61, new element=0 ("new element/subarray"), index=w64) -> (w63:i32[])
                  n34 = property on="Button Retest" class="Bool"("DisabledEnum"=w69) -> ()  [unwired: 2 in, 2 out]
                  n35 = property on="Button Next Step" class="Bool"("DisabledEnum"=w69) -> ()  [unwired: 2 in, 2 out]
                  n36 = property on="Break Point Line" class="DigNum (strict)"("DisabledEnum"=w69) -> ()  [unwired: 2 in, 2 out]
                  n37 = global write "Global Variable.vi" "Simbol Array"(w63) -> ()
                  n38 = property on="Test Sequencer" class="MCListbox (strict)"("ItemSyms"=w63) -> ()  [unwired: 2 in, 2 out]
                }
                frame True {
                  w72 = T18."Enabled" ("Disabled")
                  n39 = local write "Auto\nRestart"(u16 1 ("Auto\nRestart")) -> ()
                  n40 = local write "Report Auto"(FALSE ("Report Auto")) -> ()
                  n41 = property on="Button Retest" class="Bool"("DisabledEnum"=w72) -> ()  [unwired: 2 in, 2 out]
                  n42 = property on="Button Next Step" class="Bool"("DisabledEnum"=w72) -> ()  [unwired: 2 in, 2 out]
                  n43 = property on="Break Point Line" class="DigNum (strict)"("DisabledEnum"=w72) -> ()  [unwired: 2 in, 2 out]
                }
              }
              n44 = in-place {
                # "Test TIME Calculate"
                n45 = global read "Global Variable.vi" "Test Stop Time"() -> (w52:u32)
                n46 = global read "Global Variable.vi" "Test Start Time"() -> (w51:u32)
                n47 = Subtract(x=w52, y=w51) -> (x-y=w55:u32)
                n48 = To Double Precision Float(number=w55) -> (double precision float=w54:dbl)
                n49 = Divide(x=w54, y=u32 1000) -> (x/y=w53:dbl)
                n50 = To Unsigned Long Integer(number=w53) -> (unsigned 32bit integer=w47:u32)
                n51 = global write "Global Variable.vi" "Test Time"(w47) -> ()
                n52 = Quotient & Remainder(x=w47, y=59) -> (x-y*floor(x/y)=w45:u32, floor(x/y)=w50:u32)
                n53 = Format Into String(format string="%2dm : %2ds", w50, w45) -> (resulting string=w46:string)  [unwired: 2 in, 1 out]
                n54 = property on="Test Time" class="Str"("Value"=w46) -> ()  [unwired: 2 in, 2 out]
              }
              n55 = in-place {
                # "Date/Time"
                n56 = Get Date/Time String() -> (date string=w59:string, time string=w60:string)  [unwired: 3 in]
                n57 = Concatenate Strings(w59, " - " ("string"), w60) -> (→"Date Time":string)
              }
            }
            frame #1 {
              n58 = local read "Tab Edit/Run"() -> (w73:enum32{"Edit", "Run"})
              n59 = case shown="\"Run\"" w73 {
                frame "Edit", Default {
                }
                frame "Run" {
                  w75 = FALSE ("Delay 1S")
                  n60 = property on="Delay 1S" class="Bool (strict)"("Value"=w75) -> (error out=w76:errorcluster)  [unwired: 2 in, 1 out]
                  n61 = property on="Debugging" class="Bool (strict)"("Value"=w75) -> (error out=w74:errorcluster)  [unwired: 2 in, 1 out]
                  n62 = call <userlib>:"Clear All Errors__ogtk.vi"("Error In"=w76) -> ()  [unwired: 3 in, 1 out]
                  n63 = call <userlib>:"Clear All Errors__ogtk.vi"("Error In"=w74) -> ()  [unwired: 3 in, 1 out]
                }
              }
            }
          }
        }
        event "Barcode\nDefault": Value Change {
          n64 = event-data() -> ("NewVal"=w77:bool)  [unwired: 1 in, 5 out]
          n65 = case shown="True" w77 {
            frame False {
              n66 = property on="Barcode" class="Str"("Value"="", "Key Focus"=TRUE) -> ()  [unwired: 2 in, 2 out]
            }
            frame True {
              n67 = property on="Barcode" class="Str"("Value"="ADB-12345") -> ()  [unwired: 2 in, 2 out]
            }
          }
        }
        event "Dev INI": Value Change {
          w86 = u32 12369084
          n68 = event-data() -> ()  [unwired: 1 in, 6 out]
          n69 = in-place {
            # "Set Color of all Row to White (Devices)"
            n70 = for {
              N: 15 -> [_]
              i -> [w115]
              n71 = for {
                N: 8 -> [_]
                tunnel: w115 -> [w119]
                i -> [w120]
                n72 = Bundle By Name(cluster=T15 {"Row"=0, "Column"=0} ("Active Cell:Active Cell"), "Row"=w119, "Column"=w120) -> (w118:T15)
                n73 = property on="Box Devices" class="MCListbox (strict)"("ActiveCell"=w118, "CellBG"=u32 16448250) -> ()  [unwired: 2 in, 2 out]
              }
            }
          }
          n74 = Bundle(w86, w86) -> (w84:cluster{u32, u32})  [unwired: 1 in]
          n75 = Build Array(w84) -> (w85:cluster{u32, u32}[])
          n76 = property on="Dev INI OK?" class="Bool (strict)"("Colors [4]"=w85, "Value"=TRUE ("Dev INI OK?")) -> ()  [unwired: 2 in, 2 out]
          n77 = in-place {
            # "Clear Device Table"
            n78 = Initialize Array("", 15 ("dimension size"), 8 ("dimension size")) -> (w111:string[][])
            n79 = property on="Box Devices" class="MCListbox (strict)"("ItemNames"=w111, "TopLeft"=T14 {"Row"=0, "Column"=0} ("Top Left Visible Cell")) -> ()  [unwired: 2 in, 2 out]
          }
          n80 = call <vilib>:"Application Directory.vi"() -> ("Application Directory"=w90:path)
          n81 = Build Path(base path=w90, name or relative path="INI\\DeviceConfig.ini") -> (appended path=w88:path)
          n82 = call <vilib>:"Check if File or Folder Exists.vi"("path"=w88) -> ("error out"=w91:errorcluster, "file or folder exists?"=w87:bool)  [unwired: 8 in, 1 out]
          n83 = local write "Device INI Config File Path"(w88) -> ()
          n84 = local write "File Exist?"(w87) -> ()
          n85 = case shown="True" w87 {
            tunnel: w91 -> [w101 w108]
            tunnel: [w103 w108] -> w99
            tunnel: [0 0 ("index")] -> w82
            frame False {
              n86 = Bundle By Name(cluster=w101, "status"=TRUE, "code"=-100, "source"="Ini File not found!") -> (w103:errorcluster)
              n87 = One Button Dialog(message="File DevConfig.ini missing!") -> ()  [unwired: 1 in, 1 out]
            }
            frame True {
            }
          }
          n88 = call <vilib>:"Open Config Data.vi"("error in (no error)"=w99, "configuration file path"=w88) -> ("error out"=w95:errorcluster, "refnum"=w94:T19)  [unwired: 7 in, 1 out]
          n89 = global read "Global Variable.vi" "Array Errors"() -> (w97:errorcluster[])
          n90 = call <vilib>:"Get Section Names.vi"("error in (no error)"=w95, "refnum"=w94) -> ("error out"=w92:errorcluster, "section names"=w96:string[], "refnum out"=w93:T19)  [unwired: 7 in]
          n91 = call <vilib>:"Close Config Data.vi"("error in (no error)"=w92, "refnum"=w93) -> ()  [unwired: 8 in, 2 out]
          n92 = global write "Global Variable.vi" "Dev List"(w96) -> ()
          n93 = Replace Array Subset(array=w97, new element=w99, index=w82) -> (w98:errorcluster[])
          n94 = global write "Global Variable.vi" "Array Errors"(w98) -> ()
          n95 = global write "Global Variable.vi" "System Status"(T1."INI Devices" ("System Status")) -> ()
        }
        event "Application Quit": Value Change {
          n96 = event-data() -> ()  [unwired: 1 in, 6 out]
          n97 = flat-sequence {
            tunnel: w123 -> [w125]
            tunnel: w122 -> [w124]
            frame #0 {
              n98 = Flush Queue(queue=w125, error in (no error)=w124) -> (queue out=w127:refnum<queue>, error out=w126:errorcluster)  [unwired: 1 out]
              n99 = Release Queue(queue=w127, error in (no error)=w126) -> ()  [unwired: 1 in, 3 out]
            }
            frame #1 {
              # "Close All Ports"
              n100 = global read "Global Variable.vi" "COM Port RFID"() -> (w134:refnum<visa-resource-name>)
              n101 = global read "Global Variable.vi" "FTDI RS232 Handle"() -> (w135:u32)
              n102 = global read "Global Variable.vi" "PicoScope Handle"() -> (w129:u32)
              n103 = global read "Global Variable.vi" "FTDI RS232 Handle  RFID"() -> (w128:u32)
              n104 = global read "Global Variable.vi" "FTDI SPI Handle"() -> (w136:u32)
              n105 = global read "Global Variable.vi" "Array Errors"() -> (w132:errorcluster[])
              n106 = VISA Close(VISA resource name=w134) -> (error out=w131:errorcluster)  [unwired: 1 in]
              n107 = Replace Array Subset(array=w132, new element=w131, index=7) -> (w133:errorcluster[])
              n108 = call "FTDI SPI Close.vi"("Handler In"=w136) -> ()  [unwired: 10 in, 1 out]
              n109 = call "FT_Close_Device.vi"("Handle"=w135) -> ()  [unwired: 1 out]
              n110 = global write "Global Variable.vi" "Array Errors"(w133) -> ()
              n111 = call "PicoScope2000aClose.vi"("handle"=w129) -> ()
              n112 = call "FT_Close_Device.vi"("Handle"=w128) -> ()  [unwired: 1 out]
            }
            frame #2 {
            }
            frame #3 {
              w137 = FALSE ("stop? (T)")
              n113 = Not(x=w137) -> (.not. x?=w138:bool)
              n114 = Stop(stop? (T)=w137) -> ()
              n115 = Quit LabVIEW(quit? (T)=w138) -> ()
            }
          }
        }
        event "Run Test": Value Change {
          w148 = u32 0 ("Row")
          w140 = u32 0 ("Active Lines Cnt")
          n116 = event-data() -> ()  [unwired: 1 in, 6 out]
          n117 = global write "Global Variable.vi" "Active Lines Cnt"(w140) -> ()
          n118 = global write "Global Variable.vi" "Report Active Lines Cnt"(w140) -> ()
          n119 = global write "Global Variable.vi" "Report Step Nmb"(w140) -> ()
          n120 = global write "Global Variable.vi" "Test Time"(w140) -> ()
          n121 = local write "Restart Cnt"(w140) -> ()
          n122 = Flush Queue(queue=w152, error in (no error)=w151) -> (queue out=w145:refnum<queue>, error out=w144:errorcluster)  [unwired: 1 out]
          n123 = Bundle By Name(cluster=T14 {"Row"=0, "Column"=0} ("Top Left Visible Cell"), "Row"=w148) -> (w149:T14)
          n124 = property on="Test Sequencer Run" class="MCListbox (strict)"("TopLeft"=w149, "Value"=w148) -> ()  [unwired: 2 in, 2 out]
          n125 = property on="Test Sequencer" class="MCListbox (strict)"("TopLeft"=w149, "Value"=w148) -> ()  [unwired: 2 in, 2 out]
          n126 = local write "Enter STEP"(u32 0 ("Active Lines Cnt")) -> ()
          n127 = global read "Sequencer Array.vi" "SEQUENCER Array"() -> (w146:T16[])
          n128 = local read "Debugging"() -> (w147:bool)
          n129 = Array Size(array=w146) -> (size(s)=w142:i32)
          n130 = case shown="True" w147 {
            tunnel: w145 -> [w184 w191]
            tunnel: w144 -> [w183 w190]
            tunnel: w142 -> [w182 _]
            frame False {
              n131 = for {
                N: w182 -> [_]
                tunnel: w184 -> [w187]
                tunnel: w183 -> [w186]
                i -> [w185]
                n132 = Enqueue Element(queue=w187, element=w185, error in (no error)=w186) -> ()  [unwired: 1 in, 3 out]
              }
            }
            frame True {
              n133 = local read "Break Point Line"() -> (w188:u32)
              n134 = Increment(x=w188) -> (x+1=w189:u32)
              n135 = for {
                N: w189 -> [_]
                tunnel: w191 -> [w194]
                tunnel: w190 -> [w193]
                i -> [w192]
                n136 = Enqueue Element(queue=w194, element=w192, error in (no error)=w193) -> ()  [unwired: 1 in, 3 out]
              }
            }
          }
          n137 = for {
            N: w142 -> [_]
            i -> [w162]
            n138 = property on="Test Squencer Edit" class="MCListbox (strict)"() -> ("ItemNames"=w170:string[][])  [unwired: 2 in, 2 out]
            n139 = Bundle By Name(cluster=T15 {"Row"=0, "Column"=0} ("Active Cell:Active Cell"), "Row"=w162, "Column"=5) -> (w165:T15)
            n140 = Replace Array Subset(array=w170, new element #1="Idle", index (row) #1=w162, index (col) #1=5 ("disabled index (col)"), new element #2="", index (row) #2=w162, index (col) #2=3 ("disabled index (col)")) -> (w169:string[][])
            n141 = property on="Test Squencer Edit" class="MCListbox (strict)"("ItemNames"=w169, "ActiveCell"=w165, "CellFontColor"=u32 16448250) -> ()  [unwired: 2 in, 2 out]
          }
          n142 = control-ref of="Test Sequencer Run"() -> (w143:refnum<vi>)
          n143 = in-place {
            in-place-border: w143 -> [w172]
            in-place-border: w142 -> [w171]
            # "Set Color of all Row on Report Table"
            n144 = for {
              N: w171 -> [_]
              tunnel: w172 -> [w173]
              i -> [w174]
              n145 = for {
                N: 7 -> [_]
                tunnel: w174 -> [w179]
                tunnel: w173 -> [w176]
                i -> [w180]
                n146 = Bundle By Name(cluster=T15 {"Row"=0, "Column"=0} ("Active Cell:Active Cell"), "Row"=w179, "Column"=w180) -> (w178:T15)
                n147 = property on="Property Node" class="MCListbox (strict)"(reference=w176, "ActiveCell"=w178, "CellBG"=u32 16448250) -> ()  [unwired: 1 in, 2 out]
              }
            }
          }
          n148 = in-place {
            in-place-border: w143 -> [w159]
            in-place-border: w142 -> [w158]
            n149 = Initialize Array("", w158, 7 ("dimension size")) -> (w157:string[][])
            n150 = property on="Property Node" class="MCListbox (strict)"(reference=w159, "ItemNames"=w157, "TopLeft"=T14 {"Row"=0, "Column"=0} ("Top Left Visible Cell"), "Value"=T11 0 ("Test Sequencer")) -> ()  [unwired: 1 in, 2 out]
          }
          n151 = global write "Global Variable.vi" "System Status"(T1."START Sequencer" ("System Status")) -> ()
        }
        event "Limits": Value Change {
          n152 = event-data() -> ("OldVal"=w198:cluster{dbl, dbl, dbl}, "NewVal"=w197:cluster{dbl, dbl, dbl})  [unwired: 1 in, 4 out]
          n153 = case shown="True" FALSE {
            tunnel: w198 -> [_ w211]
            tunnel: w197 -> [_ w210]
            frame False {
            }
            frame True {
              # "max"
              # "nom"
              # "min"
              n154 = Unbundle(w211) -> (w206:dbl, w204:dbl, →"Nom Old":dbl)
              "Min Old" <- w206
              "Max Old" <- w204
              n155 = Unbundle(w210) -> (w199:dbl, w200:dbl, w205:dbl)
              "Min New" <- w199
              "Max New" <- w200
              "Nom New" <- w205
              n156 = Greater?(x=w205, y=w204) -> (0:w203:bool)
              n157 = Less?(x=w205, y=w206) -> (x < y?=w207:bool)
              n158 = case shown="True" w207 {
                tunnel: [w216 w219] -> w201
                frame False {
                  n159 = property on="Nom New" class="DigNum (strict)"() -> ("Value"=w216:dbl)  [unwired: 2 in, 2 out]
                }
                frame True {
                  n160 = property on="Min Old" class="DigNum (strict)"() -> ("Value"=w218:dbl)  [unwired: 2 in, 2 out]
                  n161 = Add(x=w218, y=0.01) -> (x+y=w219:dbl)
                }
              }
              n162 = case shown="True" w203 {
                tunnel: [w212 w213] -> w202
                tunnel: w201 -> [w212 _]
                frame False {
                }
                frame True {
                  n163 = property on="Max Old" class="DigNum (strict)"() -> ("Value"=w215:dbl)  [unwired: 2 in, 2 out]
                  n164 = Subtract(x=w215, y=0.01) -> (x-y=w213:dbl)
                }
              }
              n165 = Bundle(w199, w200, "Value"=w202) -> (w208:cluster{dbl, dbl, "Value":dbl})  [unwired: 1 in]
              n166 = property on="Limits" class="Slide (strict)"("Value"=w208) -> ()  [unwired: 2 in, 2 out]
            }
          }
          n167 = Wait (ms)(milliseconds to wait=u32 1) -> ()  [unwired: 1 out]
        }
        event "Edit Sequenser": Value Change {
          n168 = event-data() -> ()  [unwired: 1 in, 6 out]
          n169 = property on="Tab Control Main" class="TabCtl (strict)"("Value"=T2."Sequencer " ("Tab Control Main")) -> ()  [unwired: 2 in, 2 out]
        }
        event Double Click {
          n170 = event-data() -> ("Row"=w221:i32)  [unwired: 1 in, 8 out]
          n171 = flat-sequence {
            tunnel: w221 -> [w226]
            tunnel: [w223] -> w222
            tunnel: w222 -> [w237]
            frame #0 {
              n172 = global read "Sequencer Array.vi" "SEQUENCER Array"() -> (w229:T16[])
